vi "Write To Log File.vi"(8 "error in":errorcluster, 10 "log text":string, 11 "file path":path) -> (0 "error out":errorcluster)   [LabVIEW 2020, in "CICD.lvlib"]
uses:
  CICD.lvlib
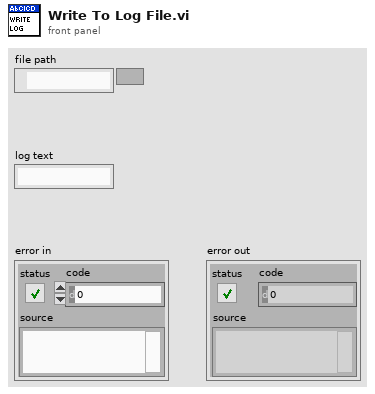
[diagram p1: front panel]
types:
  T1 = enum16{"open", "replace", "create", "open or create", "replace or create", "replace or create with confirmation"}
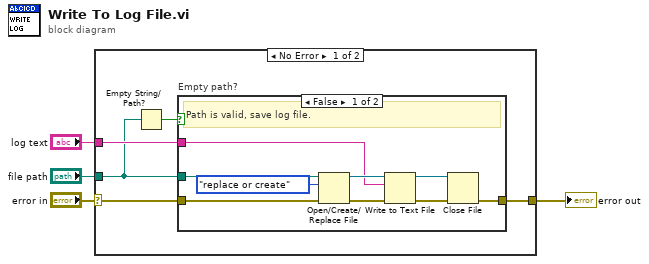
[diagram p0: block diagram]
diagram:
  n1 = case shown="No Error" "error in" {
    selector: "error in" -> [w5 w20]
    tunnel: [w9 w20] -> w4
    tunnel: "log text" -> [w8 _]
    tunnel: "file path" -> [w6 _]
    frame No Error {
      n2 = Empty String/Path?(string/path=w6) -> (empty?=w7:bool)
      n3 = case "Empty path?" shown="False" w7 {
        tunnel: w5 -> [w18 w19]
        tunnel: [w17 w19] -> w9
        tunnel: w6 -> [w16 _]
        tunnel: w8 -> [w11 _]
        frame False {
          # "Path is valid, save log file."
          n4 = Open/Create/Replace File(file path (use dialog)=w16, error in=w18, operation (0:open)=T1."replace or create") -> (refnum out=w13:refnum<file>, error out=w15:errorcluster)  [unwired: 3 in, 1 out]
          n5 = Write to Text File(file (use dialog)=w13, text=w11, error in=w15) -> (refnum out=w12:refnum<file>, error out=w14:errorcluster)  [unwired: 1 in, 1 out]
          n6 = Close File(refnum=w12, error in=w14) -> (error out=w17:errorcluster)  [unwired: 1 out]
        }
        frame True {
          # "Empty path, do nothing."
        }
      }
    }
    frame Error {
    }
  }
  "error out" <- w4
